vi "MakePythonArgumentList.vi"(1 "Arg 6":string, 2 "Arg 5":string, 3 "Arg 4":string, 4 "Arg 3":string, 5 "Arg 2":string, 6 "Arg 1":string) -> (0 "Args Out":string)   [LabVIEW 2014]
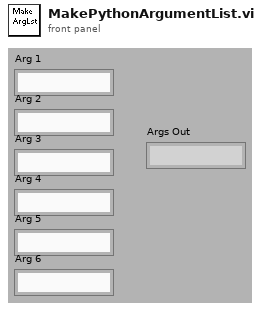
[diagram p1: front panel]
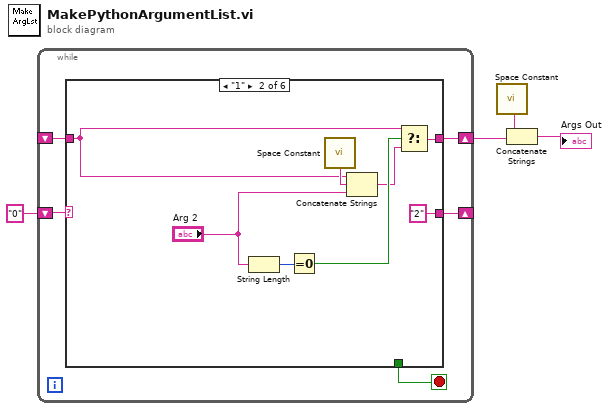
[diagram p0: block diagram]
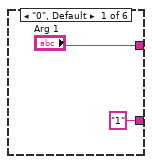
[diagram p2: hidden frame]
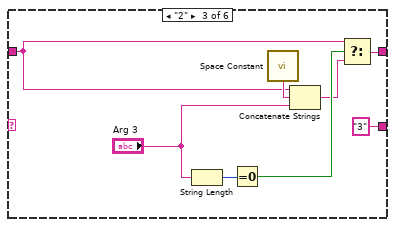
[diagram p3: hidden frame]
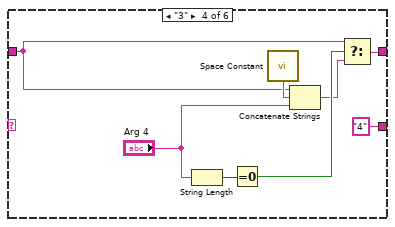
[diagram p4: hidden frame]
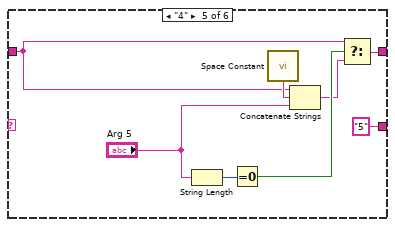
[diagram p5: hidden frame]
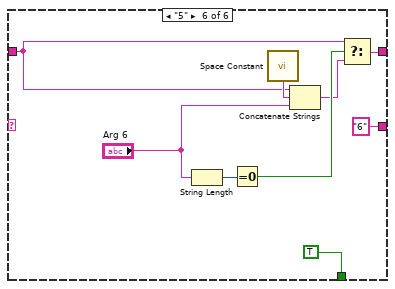
[diagram p6: hidden frame]
diagram:
  n1 = while {
    shift-right: [w5] -> _
    shift-left: "0" -> [w9]
    shift-right: [w8] -> w1
    shift-left: _ -> [w6]
    stop <- w7 stop-if-true
    n2 = case shown="\"1\"" w9 {
      tunnel: ["Arg 1" w15 w23 w31 w39 w48] -> w8
      tunnel: [_ _ _ _ _ TRUE] -> w7
      tunnel: w6 -> [_ w13 w21 w29 w37 w46]
      tunnel: ["1" "2" "3" "4" "5" "6"] -> w5
      frame "0", Default {
      }
      frame "1" {
        n3 = String Length(string="Arg 2") -> (length=w18:i32)
        n4 = Equal To 0?(x=w18) -> (x = 0?=w19:bool)
        n5 = call <vilib>:"Space Constant.vi"() -> ("String"=w17:string)
        n6 = Concatenate Strings(w13, w17, "Arg 2") -> (w14:string)
        n7 = Select(t=w13, s=w19, f=w14) -> (s? t:f=w15:string)
      }
      frame "2" {
        n8 = String Length(string="Arg 3") -> (length=w26:i32)
        n9 = Equal To 0?(x=w26) -> (x = 0?=w27:bool)
        n10 = call <vilib>:"Space Constant.vi"() -> ("String"=w25:string)
        n11 = Concatenate Strings(w21, w25, "Arg 3") -> (w22:string)
        n12 = Select(t=w21, s=w27, f=w22) -> (s? t:f=w23:string)
      }
      frame "3" {
        n13 = String Length(string="Arg 4") -> (length=w34:i32)
        n14 = Equal To 0?(x=w34) -> (x = 0?=w35:bool)
        n15 = call <vilib>:"Space Constant.vi"() -> ("String"=w33:string)
        n16 = Concatenate Strings(w29, w33, "Arg 4") -> (w30:string)
        n17 = Select(t=w29, s=w35, f=w30) -> (s? t:f=w31:string)
      }
      frame "4" {
        n18 = String Length(string="Arg 5") -> (length=w42:i32)
        n19 = Equal To 0?(x=w42) -> (x = 0?=w43:bool)
        n20 = call <vilib>:"Space Constant.vi"() -> ("String"=w41:string)
        n21 = Concatenate Strings(w37, w41, "Arg 5") -> (w38:string)
        n22 = Select(t=w37, s=w43, f=w38) -> (s? t:f=w39:string)
      }
      frame "5" {
        n23 = String Length(string="Arg 6") -> (length=w51:i32)
        n24 = Equal To 0?(x=w51) -> (x = 0?=w52:bool)
        n25 = call <vilib>:"Space Constant.vi"() -> ("String"=w50:string)
        n26 = Concatenate Strings(w46, w50, "Arg 6") -> (w47:string)
        n27 = Select(t=w46, s=w52, f=w47) -> (s? t:f=w48:string)
      }
    }
  }
  n28 = call <vilib>:"Space Constant.vi"() -> ("String"=w3:string)
  n29 = Concatenate Strings(w3, w1) -> (→"Args Out":string)
